vi "Read.vi"(8 "error in (no error)":errorcluster, 11 "ConvertTo in":refnum<class "ConvertTo_Binary.lvclass">) -> (0 "error out":errorcluster, 2 "Value":string, 3 "ConvertTo out":refnum<class "ConvertTo_Binary.lvclass">)   [LabVIEW 2021, in "ConvertTo_Binary.lvclass"]
uses:
  ConvertTo_Binary.lvclass
  ConvertTo_Binary.lvclass/ConvertTo_Binary.ctl
  Properties/Read Value.vi
  Properties/Write Value.vi
  Abs_Types/Value/Abs_Value.lvclass
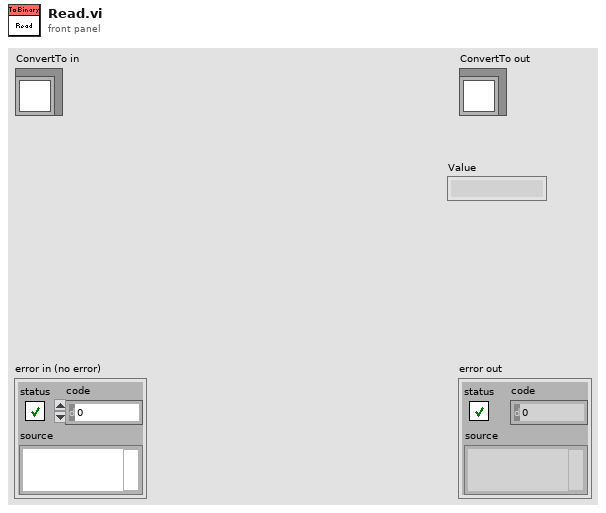
[diagram p1: front panel]
types:
  T1 = enum16{"big-endian, network order", "native, host order", "little-endian"}
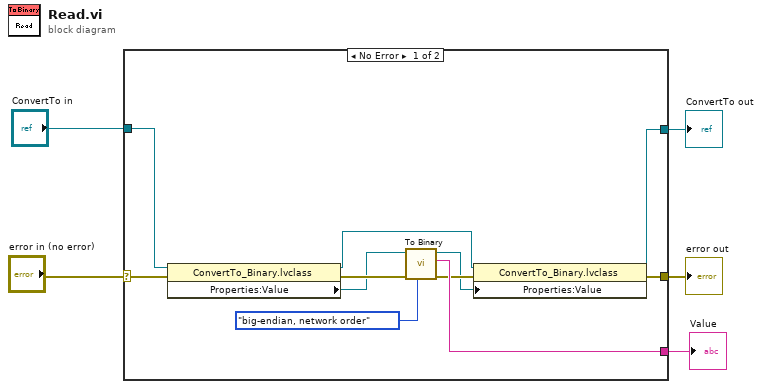
[diagram p0: block diagram]
diagram:
  n1 = case shown="No Error" "error in (no error)" {
    selector: "error in (no error)" -> [w16 w17]
    tunnel: "ConvertTo in" -> [w15 w18]
    tunnel: [w12 _] -> w3
    tunnel: [w8 w17] -> w2
    tunnel: [w7 w18] -> w1
    frame No Error {
      n2 = property class="ConvertTo_Binary.lvclass"(reference=w15, error in=w16) -> (reference out=w11:refnum<class "ConvertTo_Binary.lvclass">, error out=w14:errorcluster, "Properties:Value"=w13:refnum<class "Abs_Value.lvclass">)
      n3 = call-dynamic "To Binary.vi"("byte order"=T1."big-endian, network order", "error in (no error)"=w14, "Type in"=w13) -> ("error out"=w10:errorcluster, "Binary"=w12:string, "Type out"=w9:refnum<class "Abs_Value.lvclass">)  [unwired: 6 in]
      n4 = property class="ConvertTo_Binary.lvclass"(reference=w11, error in=w10, "Properties:Value"=w9) -> (reference out=w7:refnum<class "ConvertTo_Binary.lvclass">, error out=w8:errorcluster)
    }
    frame Error {
    }
  }
  "error out" <- w2
  "ConvertTo out" <- w1
  "Value" <- w3
